vi "Init CAN.vi"(0 "Configuration Array":T1[](array[typedef])=[{"ID"=0, "Master ID"=0, "Control Mode"=enum."Percent VBus", "Invert?"=FALSE, "Name"="Compressor"}, {"ID"=10, "Master ID"=0, "Control Mode"=enum."Percent VBus", "Invert?"=TRUE, "Name"="Left Drive"}, {"ID"=11, "Master ID"=10, "Control Mode"=enum."Percent VBus", "Invert?"=TRUE, "Name"=""}, {"ID"=12, "Master ID"=10, "Control Mode"=enum."Percent VBus", "Invert?"=TRUE, "Name"=""}, {"ID"=20, "Master ID"=0, "Control Mode"=enum."Percent VBus", "Invert?"=FALSE, "Name"="Right Drive"}, {"ID"=21, "Master ID"=20, "Control Mode"=enum."Percent VBus", "Invert?"=FALSE, "Name"=""}, {"ID"=22, "Master ID"=20, "Control Mode"=enum."Percent VBus", "Invert?"=FALSE, "Name"=""}, {"ID"=30, "Master ID"=0, "Control Mode"=enum."Percent VBus", "Invert?"=FALSE, "Name"=""}, {"ID"=31, "Master ID"=30, "Control Mode"=enum."Percent VBus", "Invert?"=FALSE, "Name"="Intake"}, {"ID"=40, "Master ID"=0, "Control Mode"=enum."Percent VBus", "Invert?"=FALSE, "Name"="Shooter"}, {"ID"=41, "Master ID"=40, "Control Mode"=enum."Percent VBus", "Invert?"=FALSE, "Name"=""}]) -> ()   [LabVIEW 2016]
uses:
  Single Talon.ctl
  <vilib>/Rock Robotics/WPI/ThirdParty/CanMotor/TalonSRX/WPI_CANTalonSRX_APIControlMode.ctl
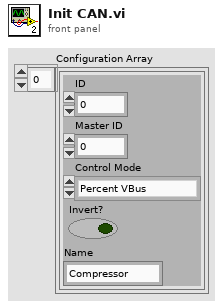
[diagram p1: front panel]
types:
  T1 = typedef "Single Talon.ctl" = cluster{"ID":i32, "Master ID":i32, "Control Mode":T2, "Invert?":bool, "Name":string}
  T2 = typedef "WPI_CANTalonSRX_APIControlMode.ctl" = enum8{"Percent VBus", "Speed", "Position", "Slave", "Unchanged / Invalid", "Voltage Compensation", "Current", "Motion Profile", "Motion Magic"}
  T3 = typedef "WPI_MotorControlDeviceRef.ctl" = cluster{"DeviceStatus":errorcluster, "Type":T4, "PWM":cluster{"PWM Channel":T5, "DeadBand":T6}, "CAN":cluster{"Device Number":u8, "SetOutput VI Ref":variant, "GetOutput VI Ref":variant, "Enable VI Ref":variant, "Disable VI Ref":variant, "Data":variant}, "Invert":bool}
  T4 = typedef "WPI_MotorControlType.ctl" = enum16{"PWM", "CAN"}
  T5 = typedef "FPGA_DIOPWMChannel.ctl" = enum8{"PWM 0", "PWM 1", "PWM 2", "PWM 3", "PWM 4", "PWM 5", "PWM 6", "PWM 7", "PWM 8", "PWM 9", "PWM MXP 0", "PWM MXP 1", "PWM MXP 2", "PWM MXP 3", "PWM MXP 4", "PWM MXP 5", "PWM MXP 6", "PWM MXP 7", "PWM MXP 8", "PWM MXP 9", "Invalid"}
  T6 = typedef "WPI_PWMDeadband.ctl" = cluster{"Name":string, "maxPositivePwm":i32, "minPositivePwm":i32, "centerPwm":i32, "maxNegativePwm":i32, "minNegativePwm":i32, "angularRange":u16}
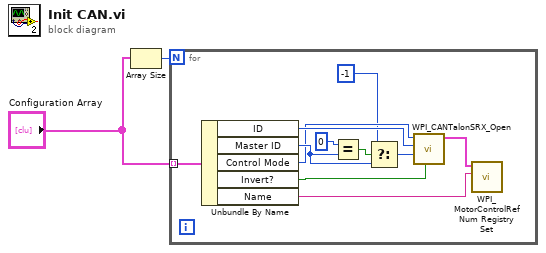
[diagram p0: block diagram]
diagram:
  n1 = Array Size(array="Configuration Array") -> (size(s)=w2:i32)
  n2 = for {
    N: w2 -> [_]
    tunnel: "Configuration Array" -> [w10] mode=indexing
    n3 = Unbundle By Name(w10) -> ("ID"=w9:i32, "Master ID"=w8:i32, "Control Mode"=w6:T2, "Invert?"=w7:bool, "Name"=w3:string)
    n4 = Equal?(x=0, y=w8) -> (x = y?=w13:bool)
    n5 = Select(t=-1, s=w13, f=w8) -> (s? t:f=w11:i32)
    n6 = call <vilib>:"WPI_CANTalonSRX_Open.vi"("Invert"=w7, "Master Device Number"=w11, "Device Number"=w9, "Control Mode"=w6) -> ("CAN Talon SRX Ref"=w4:T3)  [unwired: 6 in, 1 out]
    n7 = call <vilib>:"WPI_MotorControlRefNum Registry Set.vi"("refnum name"=w3, "MotorControlDevRef"=w4) -> ()  [unwired: 8 in, 2 out]
  }
